vi "Type String.vi"(11 "Type":variant) -> (3 "Type String":string)   [LabVIEW 2020, in "FlexBlocks.lvlib"]
uses:
  FlexBlocks.lvlib
  <resource>/ChannelSupport/_ChannelScriptingSupport/_ChannelScriptingSupport.lvlib
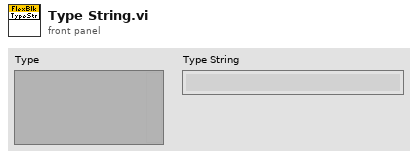
[diagram p1: front panel]
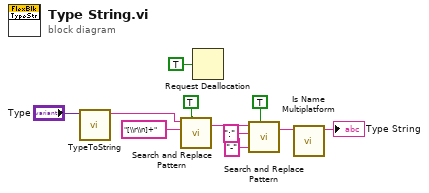
[diagram p0: block diagram]
diagram:
  n1 = call <resource>:"TypeToString.vi"("type"="Type") -> ("string"=w4:string)  [unwired: 10 in]
  n2 = call <vilib>:"Search and Replace Pattern.vi"("string"=w4, "regular expression (\"\")"="[\\r\\n]+" ("regular expression (\"\")"), "replace all? (F)"=TRUE) -> ("result string"=w8:string)  [unwired: 2 in, 1 out]
  n3 = Request Deallocation(TRUE ("flag")) -> ()
  n4 = call <vilib>:"Search and Replace Pattern.vi"("string"=w8, "regular expression (\"\")"=":" ("regular expression (\"\")"), "replace string (\"\")"="-" ("replace string (\"\")"), "replace all? (F)"=TRUE) -> ("result string"=w7:string)  [unwired: 1 in, 1 out]
  n5 = call <vilib>:"Is Name Multiplatform.vi"("filename"=w7) -> ("suggested filename"=→"Type String":string)  [unwired: 6 in, 4 out]
